vi "logEvent.vi"(8 "error in (no error)":errorcluster, 10 "New log entry":string, 11 "Text reference":refnum<vi>) -> (0 "error out":errorcluster)   [LabVIEW 2017]
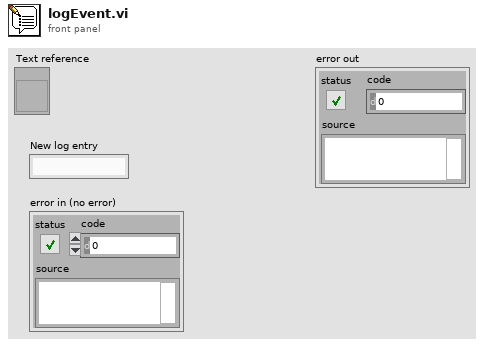
[diagram p1: front panel]
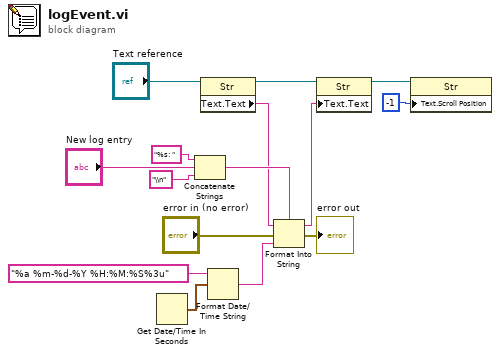
[diagram p0: block diagram]
diagram:
  n1 = Get Date/Time In Seconds() -> (seconds since 1Jan1904=w12:timestamp)
  n2 = Concatenate Strings("%s: " ("format string"), "New log entry", "\\n" ("format string")) -> (w10:string)
  n3 = property class="Str"(reference="Text reference") -> (reference out=w2:refnum<vi>, "Text.Text"=w4:string)  [unwired: 1 in, 1 out]
  n4 = Format Date/Time String(time format string (%c)="%a %m-%d-%Y %H:%M:%S%3u", seconds (now)=w12) -> (date/time string=w8:string)  [unwired: 1 in]
  n5 = Format Into String(format string=w10, initial string=w4, error in="error in (no error)", w8) -> (resulting string=w5:string, error out=→"error out":errorcluster)
  n6 = property class="Str"(reference=w2, "Text.Text"=w5) -> (reference out=w3:refnum<vi>)  [unwired: 1 in, 1 out]
  n7 = property class="Str"(reference=w3, "Text.Scroll Position"=-1) -> ()  [unwired: 1 in, 2 out]
